vi "parseXMLstring.vi"(8 "error in (no error)":errorcluster, 10 "Node Value":string, 11 "Experiment.lvclass (in)":refnum<class "Experiment.lvclass">) -> (0 "error out":errorcluster, 3 "Experiment.lvclass":refnum<class "Experiment.lvclass">)   [LabVIEW 2013, in "Experiment.lvclass"]
uses:
  Experiment.lvclass
  states.ctl
  Experiment.lvclass/Experiment.ctl
  DDS/DDS.lvclass
  HSDIO/HSDIO.lvclass
  Camera/Hamamatsu_C9100-13/Hamamatsu_C9100-13.lvclass
  Analog_output/Analog_Output.lvclass
  PI_piezo/PI_Piezo.lvclass
  Globals.vi
  <vilib>/xml/Close Reference(Node).vi
  <vilib>/xml/NI_XML.lvlib
  <resource>/objmgr/DOMUserDefRef.rc
  GPIB/GPIB.lvclass
  TCP_IP/TCP_IP.lvclass
panel:
  out "Parse Errors":string
  out "Display of element names":string[](array[string])
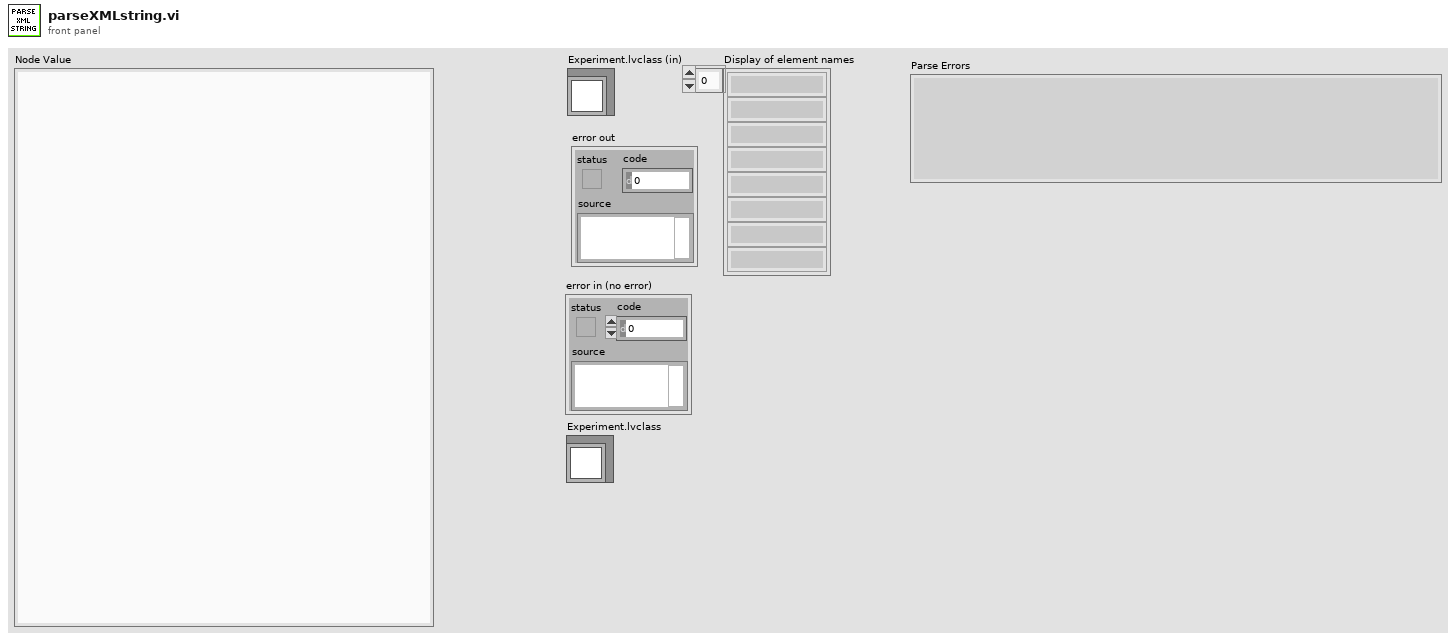
[diagram p1: front panel]
types:
  T1 = typedef "Experiment.lvclass/states.ctl" = enum16{"run", "pause", "shutdown gracefully", "halt immediately", "waiting for connection", "waiting for command"}
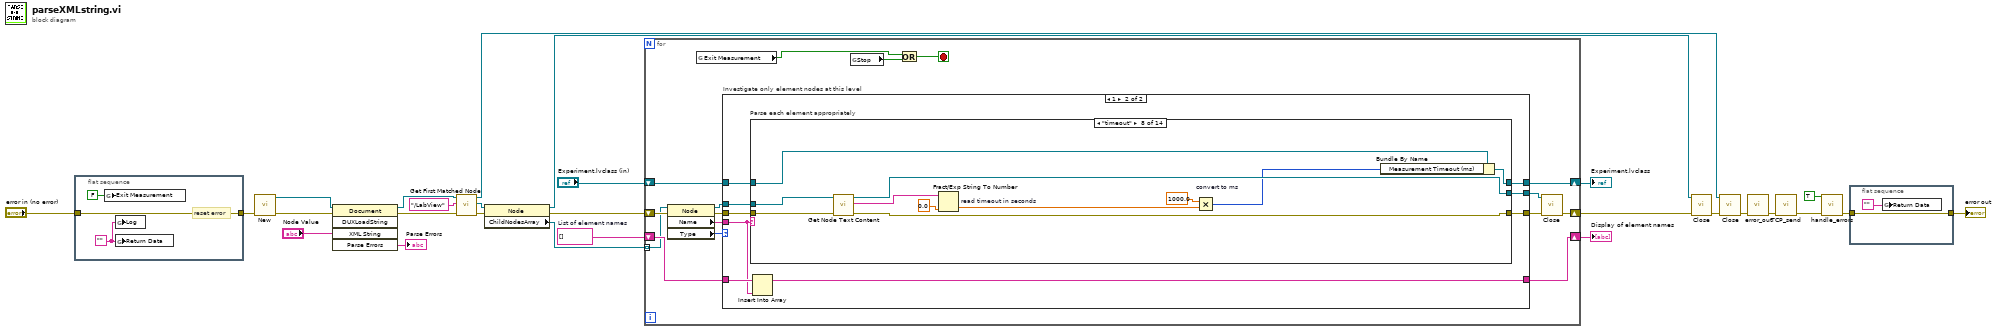
[diagram p0: block diagram]
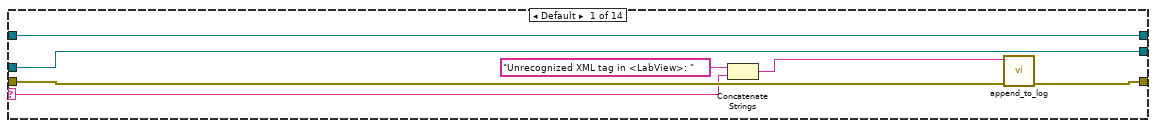
[diagram p3: hidden frame]
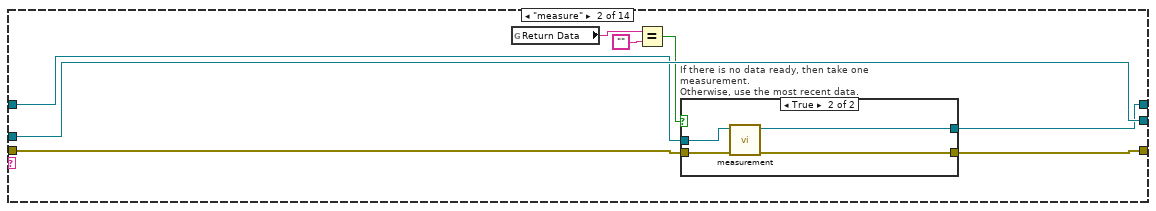
[diagram p4: hidden frame]
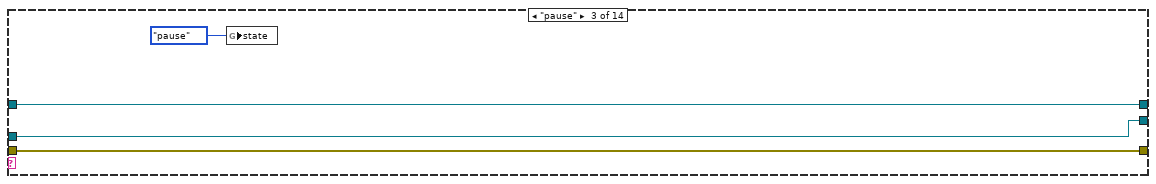
[diagram p6: hidden frame]
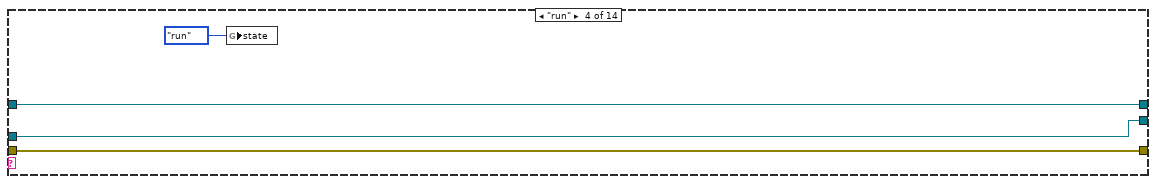
[diagram p7: hidden frame]
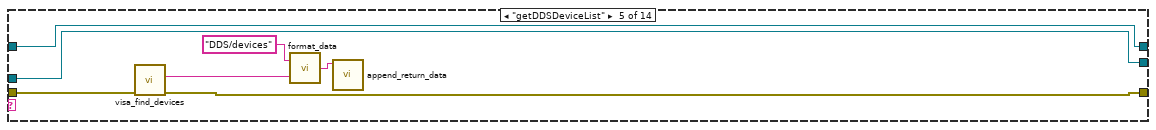
[diagram p8: hidden frame]
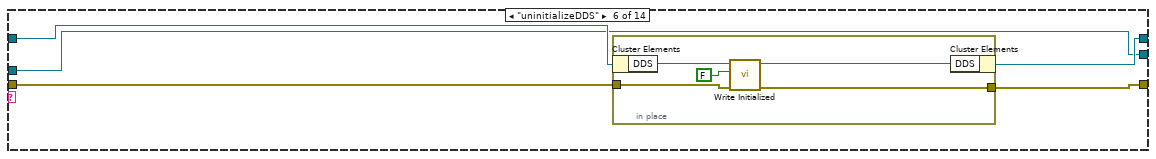
[diagram p9: hidden frame]
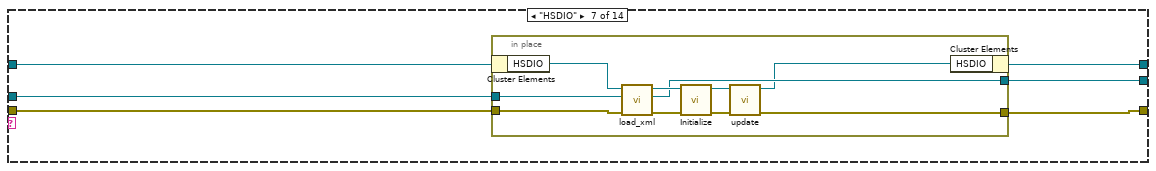
[diagram p10: hidden frame]
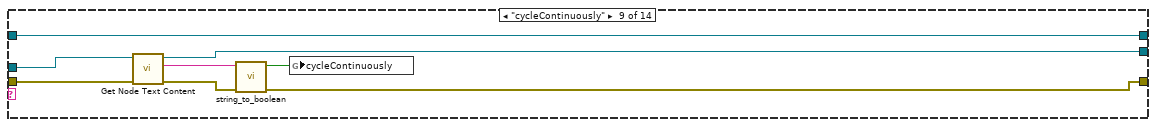
[diagram p11: hidden frame]
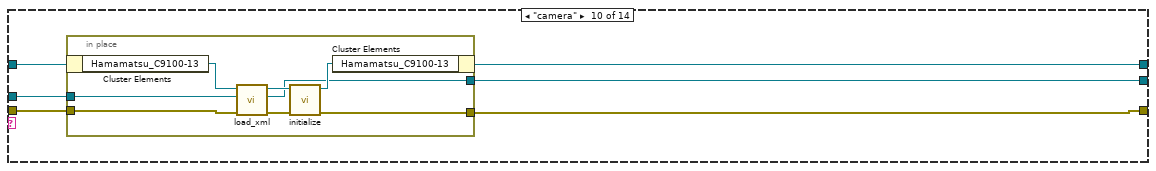
[diagram p12: hidden frame]
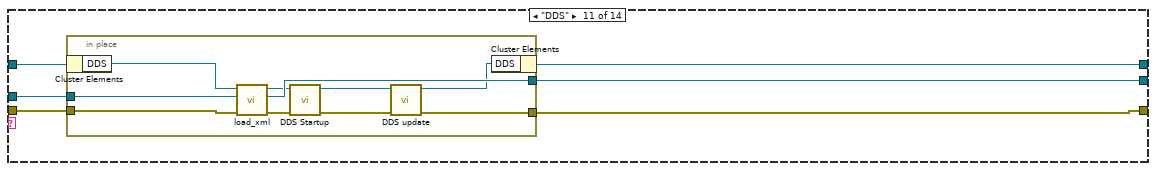
[diagram p13: hidden frame]
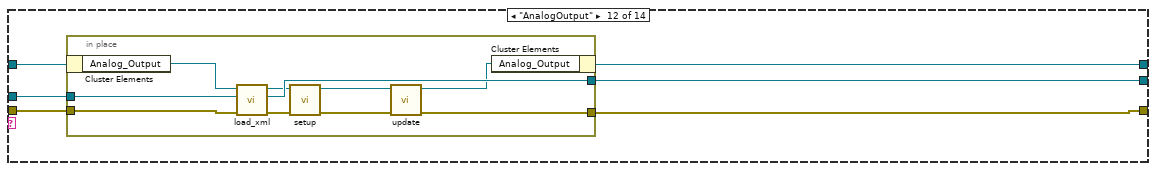
[diagram p14: hidden frame]
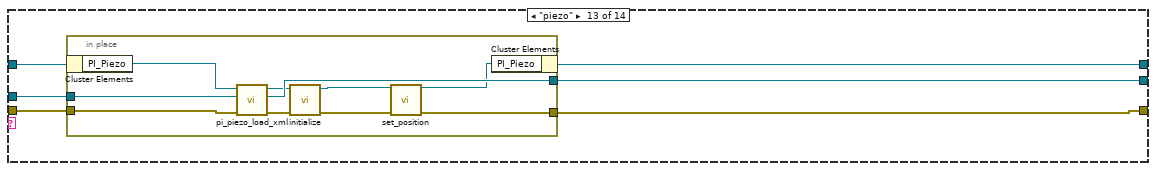
[diagram p15: hidden frame]
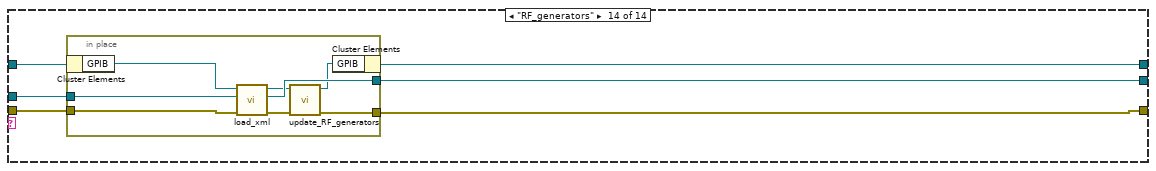
[diagram p16: hidden frame]
diagram:
  w19 = string[] []  # List of element names
  n1 = flat-sequence {
    tunnel: "error in (no error)" -> [w30]
    tunnel: [w30] -> w7
    frame #0 {
      w28 = ""
      # "reset error"
      n2 = global write "Globals.vi" "Exit Measurement"(FALSE ("Exit Measurement")) -> ()
      n3 = global write "Globals.vi" "Log"(w28) -> ()
      n4 = global write "Globals.vi" "Return Data"(w28) -> ()
    }
  }
  n5 = call <vilib>:"New.vi"("error in (no error)"=w7) -> ("error out"=w12:errorcluster, "DOM document out"=w20:refnum<k20>)  [unwired: 7 in]
  n6 = invoke class="Document" method="DUXLoadString"(reference=w20, error in=w12, "XML String"="Node Value") -> (reference out=w23:refnum<k20>, error out=w11:errorcluster, "Parse Errors"=→"Parse Errors":string)  [unwired: 2 in, 2 out]
  n7 = call <vilib>:"Get First Matched Node.vi"("error in (no error)"=w11, "XPath expression"="/LabView", "node in"=w23) -> ("error out"=w17:errorcluster, "node result"=w13:refnum<k20>, "node out"=w18:refnum<k20>)  [unwired: 6 in]
  n8 = property class="Node"(reference=w13, error in=w17) -> (reference out=w21:refnum<k20>, error out=w15:errorcluster, "ChildNodesArray"=w27:refnum<k20>[])
  n9 = for {
    tunnel: w27 -> [w40] mode=indexing
    shift-right: [w43] -> w26
    shift-left: w19 -> [w44]
    shift-right: [w42] -> w16
    shift-left: w15 -> [w41]
    shift-right: [w34] -> w9
    shift-left: "Experiment.lvclass (in)" -> [w35]
    stop <- w31 stop-if-true
    n10 = property class="Node"(reference=w40, error in=w41) -> (reference out=w37:refnum<k20>, error out=w39:errorcluster, "Name"=w45:string, "Type"=w46:i32)
    n11 = global read "Globals.vi" "Exit Measurement"() -> (w33:bool)
    n12 = case "Investigate only element nodes at this level" shown="1" w46 {
      tunnel: w45 -> [_ w57]
      tunnel: w44 -> [w50 w59]
      tunnel: [w50 w58] -> w43
      tunnel: w37 -> [w48 w56]
      tunnel: w39 -> [w49 w55]
      tunnel: [w49 w54] -> w38
      tunnel: [w48 w53] -> w36
      tunnel: w35 -> [w47 w52]
      tunnel: [w47 w51] -> w34
      frame Default {
      }
      frame 1 {
        n13 = case "Parse each element appropriately" shown="\"timeout\"" w57 {
          selector: w57 -> [w63 _ _ _ _ _ _ _ _ _ _ _ _ _]
          tunnel: w56 -> [w61 w74 w81 w85 w92 w96 w107 w131 w140 w142 w156 w172 w188 w204]
          tunnel: w55 -> [w66 w70 w82 w86 w91 w98 w109 w132 w136 w143 w157 w173 w189 w205]
          tunnel: [w65 w69 w82 w86 w90 w97 w108 w123 w135 w144 w158 w174 w190 w206] -> w54
          tunnel: [w61 w74 w81 w85 w92 w96 w106 w130 w137 w141 w155 w171 w187 w203] -> w53
          tunnel: w52 -> [w60 w68 w83 w87 w93 w100 w111 w129 w133 w146 w160 w176 w192 w208]
          tunnel: [w60 w67 w83 w87 w93 w99 w110 w122 w133 w145 w159 w175 w191 w207] -> w51
          frame Default {
            n14 = Concatenate Strings("Unrecognized XML tag in <LabView>: " ("string"), w63) -> (w62:string)
            n15 = call "append_to_log.vi"("error in"=w66, "string"=w62) -> ("error out"=w65:errorcluster)  [unwired: 9 in]
          }
          frame "measure" {
            n16 = global read "Globals.vi" "Return Data"() -> (w73:string)
            n17 = Equal?(x=w73, y="") -> (x = y?=w71:bool)
            n18 = case "If there is no data ready, then take one measurement.\nOtherwise, use the most recent data." shown="True" w71 {
              tunnel: w70 -> [w76 w80]
              tunnel: [w76 w79] -> w69
              tunnel: w68 -> [w75 w78]
              tunnel: [w75 w77] -> w67
              frame False {
              }
              frame True {
                n19 = call "measurement.vi"("error in (no error)"=w80, "Experiment.lvclass"=w78) -> ("error out"=w79:errorcluster, "Experiment out"=w77:refnum<class "Experiment.lvclass">)  [unwired: 6 in]
              }
            }
          }
          frame "pause" {
            n20 = global write "Globals.vi" "state"(states."pause" ("state")) -> ()
          }
          frame "run" {
            n21 = global write "Globals.vi" "state"(states."run" ("state")) -> ()
          }
          frame "getDDSDeviceList" {
            n22 = call "visa_find_devices.vi"("error in (no error)"=w91) -> ("error out"=w90:errorcluster, "devices found string"=w89:string)  [unwired: 8 in, 1 out]
            n23 = call "format_data.vi"("data"=w89, "name"="DDS/devices") -> ("concatenated string"=w94:string)
            n24 = call "append_return_data.vi"("Return Data"=w94) -> ()  [unwired: 11 in]
          }
          frame "uninitializeDDS" {
            n25 = in-place {
              in-place-border: w98 -> [w102]
              in-place-border: [w101] -> w97
              n26 = in-place-cluster #1(w100) -> ("DDS"=w105:refnum<class "DDS.lvclass">)
              n27 = call-dynamic "Write Initialized.vi"("error in (no error)"=w102, "Initialized"=FALSE, "DDS in"=w105) -> ("error out"=w101:errorcluster, "DDS out"=w104:refnum<class "DDS.lvclass">)  [unwired: 7 in]
              n28 = in-place-cluster #1("DDS"=w104) -> (w99:refnum<class "Experiment.lvclass">)
            }
          }
          frame "HSDIO" {
            n29 = in-place {
              in-place-border: w109 -> [w120]
              in-place-border: [w113] -> w108
              in-place-border: w107 -> [w121]
              in-place-border: [w116] -> w106
              n30 = in-place-cluster #2(w111) -> ("HSDIO"=w119:refnum<class "HSDIO.lvclass">)
              n31 = call "load_xml.vi"("error in"=w120, "child node in"=w121, "HSDIO (in)"=w119) -> ("error out"=w117:errorcluster, "child node out"=w116:refnum<k20>, "HSDIO"=w118:refnum<class "HSDIO.lvclass">)  [unwired: 6 in]
              n32 = call "Initialize.vi"("error in (no error)"=w117, "HSDIO in"=w118) -> ("error out"=w114:errorcluster, "HSDIO out"=w115:refnum<class "HSDIO.lvclass">)  [unwired: 8 in]
              n33 = call-dynamic "update.vi"("error in (no error)"=w114, "HSDIO in"=w115) -> ("error out"=w113:errorcluster, "HSDIO out"=w112:refnum<class "HSDIO.lvclass">)  [unwired: 8 in]
              n34 = in-place-cluster #2("HSDIO"=w112) -> (w110:refnum<class "Experiment.lvclass">)
            }
          }
          frame "timeout" {
            n35 = call <vilib>:"Get Node Text Content.vi"("error in (no error)"=w132, "node in"=w131) -> ("error out"=w123:errorcluster, "node text"=w127:string, "node out"=w130:refnum<k20>)  [unwired: 7 in]
            n36 = Fract/Exp String To Number "read timeout in seconds"(string=w127, default (0 dbl)=0.0 ("default (0 I32)")) -> (number=w124:dbl)  [unwired: 2 in, 1 out]
            n37 = Multiply "convert to ms"(x=1000.0, y=w124) -> (x*y=w125:u32)
            n38 = Bundle By Name(cluster=w129, "Measurement Timeout (ms)"=w125) -> (w122:refnum<class "Experiment.lvclass">)
          }
          frame "cycleContinuously" {
            n39 = call <vilib>:"Get Node Text Content.vi"("error in (no error)"=w136, "node in"=w140) -> ("error out"=w139:errorcluster, "node text"=w138:string, "node out"=w137:refnum<k20>)  [unwired: 7 in]
            n40 = call "string_to_boolean.vi"("error in"=w139, "string"=w138) -> ("error out"=w135:errorcluster, "boolean"=w134:bool)  [unwired: 8 in]
            n41 = global write "Globals.vi" "cycleContinuously"(w134) -> ()
          }
          frame "camera" {
            n42 = in-place {
              in-place-border: [w150] -> w144
              in-place-border: w143 -> [w149]
              in-place-border: w142 -> [w148]
              in-place-border: [w147] -> w141
              n43 = in-place-cluster #3(w146) -> ("Hamamatsu_C9100-13"=w153:refnum<class "Hamamatsu_C9100-13.lvclass">)
              n44 = call "load_xml.vi"("error in"=w149, "child node in"=w148, "Hamamatsu_C9100-13.lvclass (in)"=w153) -> ("error out"=w151:errorcluster, "child node out"=w147:refnum<k20>, "Hamamatsu_C9100-13.lvclass"=w152:refnum<class "Hamamatsu_C9100-13.lvclass">)  [unwired: 6 in]
              n45 = call-dynamic "initialize.vi"("error in (no error)"=w151, "Hamamatsu_C9100-13 in"=w152) -> ("error out"=w150:errorcluster, "Hamamatsu_C9100-13 out"=w154:refnum<class "Hamamatsu_C9100-13.lvclass">)  [unwired: 8 in]
              n46 = in-place-cluster #3("Hamamatsu_C9100-13"=w154) -> (w145:refnum<class "Experiment.lvclass">)
            }
          }
          frame "DDS" {
            n47 = in-place {
              in-place-border: [w165] -> w158
              in-place-border: w157 -> [w168]
              in-place-border: w156 -> [w169]
              in-place-border: [w167] -> w155
              n48 = in-place-cluster #4(w160) -> ("DDS"=w170:refnum<class "DDS.lvclass">)
              n49 = call "load_xml.vi"("error in"=w168, "child node in"=w169, "DDS.lvclass (in)"=w170) -> ("error out"=w163:errorcluster, "child node out"=w167:refnum<k20>, "DDS.lvclass"=w164:refnum<class "DDS.lvclass">)  [unwired: 6 in]
              n50 = call "DDS Startup.vi"("error in (no error)"=w163, "DDS.lvclass (in)"=w164) -> ("error out"=w162:errorcluster, "DDS.lvclass"=w161:refnum<class "DDS.lvclass">)  [unwired: 8 in]
              n51 = call "DDS update.vi"("error in (no error)"=w162, "DDS.lvclass (in)"=w161) -> ("error out"=w165:errorcluster, "DDS.lvclass"=w166:refnum<class "DDS.lvclass">)  [unwired: 8 in]
              n52 = in-place-cluster #4("DDS"=w166) -> (w159:refnum<class "Experiment.lvclass">)
            }
          }
          frame "AnalogOutput" {
            n53 = in-place {
              in-place-border: [w180] -> w174
              in-place-border: w173 -> [w184]
              in-place-border: w172 -> [w185]
              in-place-border: [w183] -> w171
              n54 = in-place-cluster #5(w176) -> ("Analog_Output"=w186:refnum<class "Analog_Output.lvclass">)
              n55 = call "load_xml.vi"("error in"=w184, "child node in"=w185, "Analog_Output.lvclass (in)"=w186) -> ("error out"=w182:errorcluster, "child node out"=w183:refnum<k20>, "Analog_Output.lvclass"=w179:refnum<class "Analog_Output.lvclass">)  [unwired: 6 in]
              n56 = call "setup.vi"("error in (no error)"=w182, "Analog_Output in"=w179) -> ("error out"=w181:errorcluster, "Analog_Output out"=w178:refnum<class "Analog_Output.lvclass">)  [unwired: 8 in]
              n57 = call-dynamic "update.vi"("error in (no error)"=w181, "Analog_Output in"=w178) -> ("error out"=w180:errorcluster, "Analog_Output out"=w177:refnum<class "Analog_Output.lvclass">)  [unwired: 8 in]
              n58 = in-place-cluster #5("Analog_Output"=w177) -> (w175:refnum<class "Experiment.lvclass">)
            }
          }
          frame "piezo" {
            n59 = in-place {
              in-place-border: [w194] -> w190
              in-place-border: w189 -> [w200]
              in-place-border: w188 -> [w201]
              in-place-border: [w199] -> w187
              n60 = in-place-cluster #6(w192) -> ("PI_Piezo"=w202:refnum<class "PI_Piezo.lvclass">)
              n61 = call "pi_piezo_load_xml.vi"("error in"=w200, "child node in"=w201, "PI_Piezo (in)"=w202) -> ("error out"=w197:errorcluster, "child node out"=w199:refnum<k20>, "PI_Piezo"=w198:refnum<class "PI_Piezo.lvclass">)  [unwired: 6 in]
              n62 = call-dynamic "initialize.vi"("error in (no error)"=w197, "PI_Piezo in"=w198) -> ("error out"=w193:errorcluster, "PI_Piezo out"=w196:refnum<class "PI_Piezo.lvclass">)  [unwired: 8 in]
              n63 = call "set_position.vi"("PI_Piezo (in)"=w196, "error in"=w193) -> ("PI_Piezo"=w195:refnum<class "PI_Piezo.lvclass">, "error out"=w194:errorcluster)  [unwired: 12 in]
              n64 = in-place-cluster #6("PI_Piezo"=w195) -> (w191:refnum<class "Experiment.lvclass">)
            }
          }
          frame "RF_generators" {
            n65 = in-place {
              in-place-border: [w213] -> w206
              in-place-border: w205 -> [w215]
              in-place-border: w204 -> [w214]
              in-place-border: [w212] -> w203
              n66 = in-place-cluster #7(w208) -> ("GPIB"=w216:refnum<class "GPIB.lvclass">)
              n67 = call "load_xml.vi"("error in"=w215, "child node in"=w214, "GPIB (in)"=w216) -> ("error out"=w211:errorcluster, "child node out"=w212:refnum<k20>, "GPIB"=w210:refnum<class "GPIB.lvclass">)  [unwired: 6 in]
              n68 = call "update_RF_generators.vi"("error in"=w211, "GPIB (in)"=w210) -> ("error out"=w213:errorcluster, "GPIB"=w209:refnum<class "GPIB.lvclass">)  [unwired: 8 in]
              n69 = in-place-cluster #7("GPIB"=w209) -> (w207:refnum<class "Experiment.lvclass">)
            }
          }
        }
        n70 = Insert Into Array(array=w59, new element=w57) -> (w58:string[])  [unwired: 1 in]
      }
    }
    n71 = global read "Globals.vi" "Stop"() -> (w32:bool)
    n72 = Or(x=w33, y=w32) -> (x .or. y?=w31:bool)
    n73 = call-poly <vilib>:"Close.vi"("error in (no error)"=w38, "node"=w36) -> ("error out"=w42:errorcluster)  [unwired: 7 in]
  }
  "Display of element names" <- w26
  "Experiment.lvclass" <- w9
  n74 = call-poly <vilib>:"Close.vi"("error in (no error)"=w16, "node"=w21) -> ("error out"=w14:errorcluster)  [unwired: 7 in]
  n75 = call-poly <vilib>:"Close.vi"("error in (no error)"=w14, "node"=w18) -> ("error out"=w5:errorcluster)  [unwired: 7 in]
  n76 = call "error_out.vi"("error in (no error)"=w5) -> ("error out"=w6:errorcluster)  [unwired: 10 in]
  n77 = call "TCP_send.vi"("error in (no error)"=w6) -> ("error out"=w4:errorcluster)  [unwired: 10 in]
  n78 = call "handle_errors.vi"("Exit Operation"=TRUE ("Exit Measurement"), "error in (no error)"=w4) -> ("error out"=w1:errorcluster)  [unwired: 13 in]
  n79 = flat-sequence {
    tunnel: [w217] -> w2
    tunnel: w1 -> [w217]
    frame #0 {
      n80 = global write "Globals.vi" "Return Data"("") -> ()
    }
  }
  "error out" <- w2
